vi "CreateCAlexHeader.vi"(8 "error in (no error)":errorcluster) -> (0 "error out":errorcluster, 1 "ColumnOfVar":i32[](array[numeric]), 2 "NumOfColumn":i32, 3 "header":string)   [LabVIEW 2015]
uses:
  Classes/CAlex2/TypeDef/LowerBodyDim.ctl
  Classes/ForceField/TypeDef/FF_Gains.ctl
  Classes/MotorControl/TypeDef/MotorMode.ctl
  <vilib>/GoldZinc Software/auzn custom VIs/CustomVI.lvlib
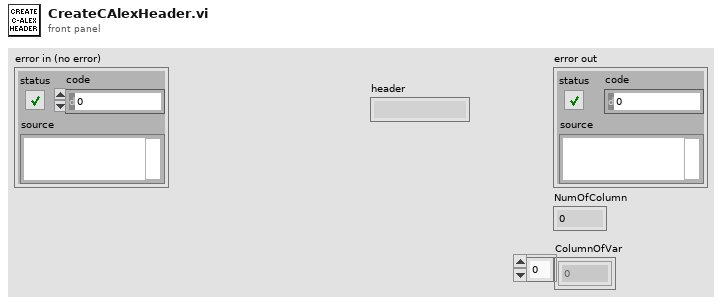
[diagram p1: front panel]
types:
  T1 = typedef "CAlex2.lvclass/LowerBodyDim.ctl" = cluster{"BodyDim":cluster{"ThighLt (m)":dbl, "ShankLt (m)":dbl, "HipWd (m)":dbl}, "BodyWt":cluster{"Thigh (kg)":dbl, "Shank (kg)":dbl}, "Cuff Loc":cluster{"HipCuffWd (m)":dbl, "HipCuffHt (m)":dbl, "HipFwdShift (m)":dbl, "ThighToKnee (m)":dbl, "ThighCuffDist (in)":dbl, "ShankToKnee (m)":dbl}}
  T2 = typedef "ForceField.lvclass/FF_Gains.ctl" = cluster{"Kn":dbl, "Dn":dbl, "Kt":dbl, "Dt":dbl, "Kd":dbl, "Ns":dbl}
  T3 = typedef "MotorControl.lvclass/MotorMode.ctl" = enum16{"Idle", "FF", "PID"}
  T4 = cluster{"ThighLt (m)":dbl, "ShankLt (m)":dbl, "HipWd (m)":dbl}
  T5 = cluster{"HipCuffWd (m)":dbl, "HipCuffHt (m)":dbl, "HipFwdShift (m)":dbl, "ThighToKnee (m)":dbl, "ThighCuffDist (in)":dbl, "ShankToKnee (m)":dbl}
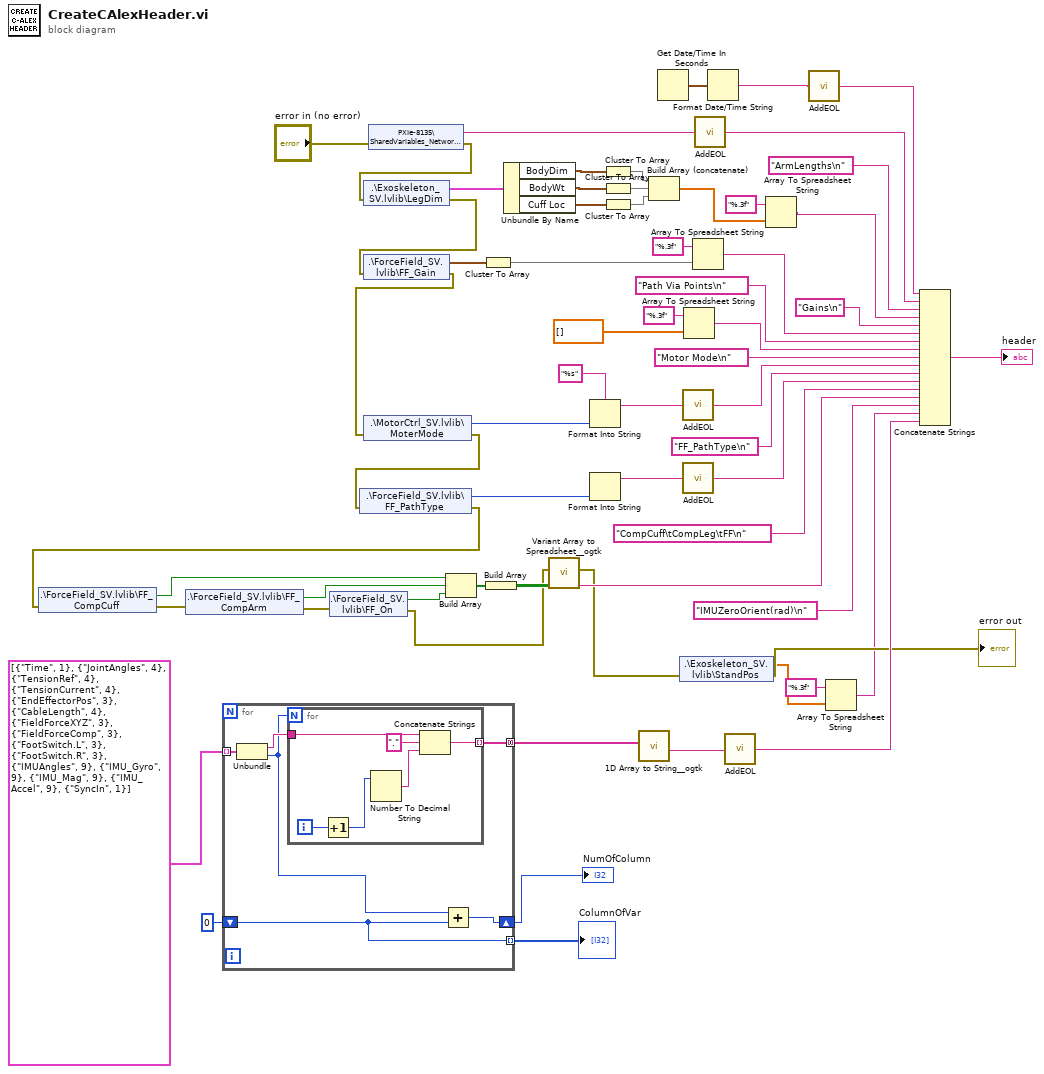
[diagram p0: block diagram]
diagram:
  n1 = for {
    tunnel: [w70] -> w52 mode=concatenating
    tunnel: cluster{string, i32}[] [{"Time", 1}, {"JointAngles", 4}, {"TensionRef", 4}, {"TensionCurrent", 4}, {"EndEffectorPos", 3}, {"CableLength", 4}, {"FieldForceXYZ", 3}, {"FieldForceComp", 3}, {"FootSwitch.L", 3}, {"FootSwitch.R", 3}, {"IMUAngles", 9}, {"IMU_Gyro", 9}, {"IMU_Mag", 9}, {"IMU_Accel", 9}, {"SyncIn", 1}] ("Array") -> [w68] mode=indexing
    shift-right: [w66] -> w15
    shift-left: 0 -> [w65]
    tunnel: [w65] -> w16 mode=indexing
    n2 = Unbundle(w68) -> (w69:string, w67:i32)
    n3 = for {
      N: w67 -> [_]
      tunnel: w69 -> [w76]
      tunnel: [w71] -> w70 mode=indexing
      i -> [w73]
      n4 = Increment(x=w73) -> (x+1=w72:i32)
      n5 = Number To Decimal String(number=w72) -> (decimal integer string=w74:string)  [unwired: 1 in]
      n6 = Concatenate Strings(w76, ".", w74) -> (w71:string)
    }
    n7 = Add(x=w67, y=w65) -> (x+y=w66:i32)
  }
  "NumOfColumn" <- w15
  "ColumnOfVar" <- w16
  n8 = shared-variable "PXIe-8135\\SharedVariables_Network.lvlib\\FileName"(error in="error in (no error)") -> (w27:string, error out=w51:errorcluster)
  n9 = shared-variable ".\\Exoskeleton_SV.lvlib\\LegDim"(error in=w51) -> (w9:T1, error out=w53:errorcluster)
  n10 = shared-variable ".\\ForceField_SV.lvlib\\FF_Gain"(error in=w53) -> (w54:T2, error out=w43:errorcluster)
  n11 = shared-variable ".\\MotorCtrl_SV.lvlib\\MoterMode"(error in=w43) -> (w55:T3, error out=w34:errorcluster)
  n12 = shared-variable ".\\ForceField_SV.lvlib\\FF_PathType"(error in=w34) -> (w32:i8, error out=w33:errorcluster)
  n13 = shared-variable ".\\ForceField_SV.lvlib\\FF_CompCuff"(error in=w33) -> (w38:bool, error out=w42:errorcluster)
  n14 = shared-variable ".\\ForceField_SV.lvlib\\FF_CompArm"(error in=w42) -> (w39:bool, error out=w41:errorcluster)
  n15 = shared-variable ".\\ForceField_SV.lvlib\\FF_On"(error in=w41) -> (w40:bool, error out=w35:errorcluster)
  n16 = Build Array(w38, w39, w40) -> (w37:bool[])
  n17 = Cluster To Array(cluster=w54) -> (array=w11:dbl[])
  n18 = Build Array(w37) -> (w36:bool[][])
  n19 = Unbundle By Name(w9) -> ("BodyDim"=w48:T4, "BodyWt"=w47:cluster{"Thigh (kg)":dbl, "Shank (kg)":dbl}, "Cuff Loc"=w46:T5)
  n20 = call <userlib>:"Variant Array to Spreadsheet__ogtk.vi"("2D Variant Array"=w36, "error in (no error)"=w35) -> ("spreadsheet string"=w31:string, "error out"=w19:errorcluster)  [unwired: 8 in]
  n21 = Format Into String(format string="%s", w55) -> (resulting string=w29:string)  [unwired: 2 in, 1 out]
  n22 = Format Into String(w32) -> (resulting string=w23:string)  [unwired: 3 in, 1 out]
  n23 = Cluster To Array(cluster=w48) -> (array=w49:dbl[])
  n24 = Cluster To Array(cluster=w47) -> (array=w45:dbl[])
  n25 = Cluster To Array(cluster=w46) -> (array=w44:dbl[])
  n26 = call <userlib>:"1D Array to String__ogtk.vi"("Array of Strings"=w52) -> ("delimited string"=w21:string)  [unwired: 10 in]
  n27 = Build Array (concatenate)(w49, w45, w44) -> (w14:dbl[])
  n28 = Get Date/Time In Seconds() -> (seconds since 1Jan1904=w60:timestamp)
  n29 = shared-variable ".\\Exoskeleton_SV.lvlib\\StandPos"(error in=w19) -> (w3:dbl[], error out=→"error out":errorcluster)
  n30 = call <vilib>:"AddEOL.vi"("String in"=w29) -> ("String+\\n"=w28:string)
  n31 = call <vilib>:"AddEOL.vi"("String in"=w23) -> ("String+\\n"=w22:string)
  n32 = Array To Spreadsheet String(array=dbl[] [] ("Data"), 3:"%.3f" ("format string")) -> (spreadsheet string=w6:string)  [unwired: 1 in]
  n33 = Array To Spreadsheet String(array=w11, 3:"%.3f" ("format string")) -> (spreadsheet string=w10:string)  [unwired: 1 in]
  n34 = call <vilib>:"AddEOL.vi"("String in"=w27) -> ("String+\\n"=w26:string)
  n35 = Format Date/Time String(seconds (now)=w60) -> (date/time string=w25:string)  [unwired: 2 in]
  n36 = call <vilib>:"AddEOL.vi"("String in"=w21) -> ("String+\\n"=w20:string)
  n37 = Array To Spreadsheet String(array=w14, 3:"%.3f" ("format string")) -> (spreadsheet string=w13:string)  [unwired: 1 in]
  n38 = call <vilib>:"AddEOL.vi"("String in"=w25) -> ("String+\\n"=w24:string)
  n39 = Array To Spreadsheet String(array=w3, 3:"%.3f" ("format string")) -> (spreadsheet string=w2:string)  [unwired: 1 in]
  n40 = Concatenate Strings(w24, w26, "ArmLengths\n" ("string"), w13, "Gains\n" ("string"), w10, "Path Via Points\n" ("string"), w6, "Motor Mode\n" ("string"), w28, "FF_PathType\n" ("string"), w22, "CompCuff\tCompLeg\tFF\n" ("string"), w31, "IMUZeroOrient(rad)\n" ("string"), w2, w20) -> (→"header":string)
